vi "Disconnect Power Supply.vi"(2 "error in":errorcluster, 3 "Power Supply Model":T1=enum."Keithley 24XX", 4 "Power Supply Address":refnum<visa-resource-name>) -> (0 "error out":errorcluster)   [LabVIEW 2020]
uses:
  Typedefs/Power Supply Models.ctl
  <instrlib>/Keithley 24XX/Keithley 24XX.lvlib
  <instrlib>/Agilent 6XXX Series/Agilent 6XXX Series.lvlib
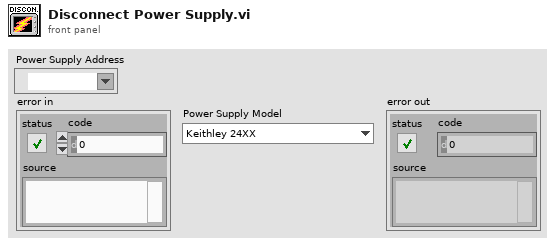
[diagram p1: front panel]
types:
  T1 = typedef "Power Supply Models.ctl" = enum16{"Keithley 248", "Keithley 237", "Keithley 24XX", "HP/Agilent 6XXX"}
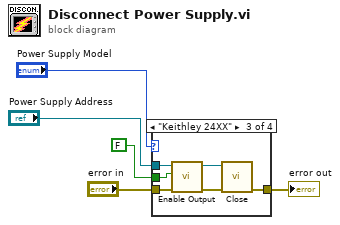
[diagram p0: block diagram]
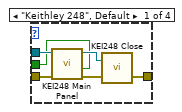
[diagram p2: hidden frame]
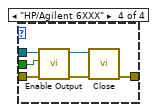
[diagram p4: hidden frame]
diagram:
  n1 = case shown="\"Keithley 24XX\"" "Power Supply Model" {
    tunnel: "Power Supply Address" -> [w10 _ w17 w23]
    tunnel: "error in" -> [w9 w12 w16 w22]
    tunnel: [w11 w12 w18 w24] -> w3
    tunnel: FALSE -> [w6 _ w13 w19]
    frame "Keithley 248", Default {
      n2 = call "KEI248 Main Panel"("Output Switch"=w6, "error in"=w9, "VISA resource name"=w10) -> ("error out"=w7:errorcluster, "VISA resource name out"=w8:refnum<visa-resource-name>)  [unwired: 5 in]
      n3 = call <instrlib>:"KEI248 Close.vi"("error in"=w7, "VISA resource name"=w8) -> ("error out"=w11:errorcluster)  [unwired: 1 in]
    }
    frame "Keithley 237" {
    }
    frame "Keithley 24XX" {
      n4 = call <instrlib>:"Enable Output.vi"("error in (no error)"=w16, "Enable Output (T: Enable)"=w13, "VISA resource name"=w17) -> ("error out"=w14:errorcluster, "VISA resource name out"=w15:refnum<visa-resource-name>)  [unwired: 7 in]
      n5 = call <instrlib>:"Close.vi"("error in (no error)"=w14, "VISA resource name"=w15) -> ("error out"=w18:errorcluster)  [unwired: 9 in]
    }
    frame "HP/Agilent 6XXX" {
      n6 = call <instrlib>:"Enable Output.vi"("error in (no error)"=w22, "output (T:on)"=w19, "VISA resource name"=w23) -> ("error out"=w21:errorcluster, "VISA resource name out"=w20:refnum<visa-resource-name>)  [unwired: 7 in]
      n7 = call <instrlib>:"Close.vi"("error in (no error)"=w21, "VISA resource name"=w20) -> ("error out"=w24:errorcluster)  [unwired: 9 in]
    }
  }
  "error out" <- w3
